vi "GOOP_Utility_IsLibVI.vi"(7 "KeepClassOpen(False)":bool, 8 "error in (no error)":errorcluster, 10 "ProjectItem":refnum<vi>, 11 "Object":u64) -> (0 "error out":errorcluster, 1 "ClassItem(If Found)":refnum<vi>, 2 "LibProvider":string, 3 "Is Lib VI?":bool)   [LabVIEW 2014]
uses:
  <resource>/Framework/Providers/Open_GDS/ClassProviders/Common/LvLib_class/GDSLvLib_LibTypeSettingNames.ctl
  <resource>/Framework/Providers/Open_GDS/ClassProviders/Provider_LvNativeClass/LvNativeProviderName.ctl
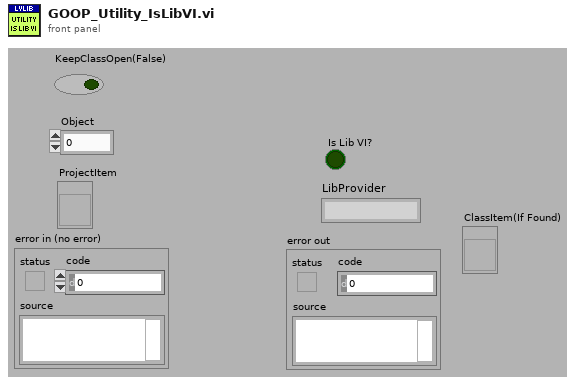
[diagram p1: front panel]
types:
  T1 = typedef "LvNativeProviderName.ctl" = enum16{"Endevo LabVIEW Native"}
  T2 = typedef "GDSLvLib_LibTypeSettingNames.ctl" = enum16{"EndevoGOOP_LibProvider", "EndevoGOOP_TemplateUsed", "EndevoGOOP_TemplateVersion", "EndevoGOOP_PlugIns", "EndevoGOOP_ConnectorPanePattern"}
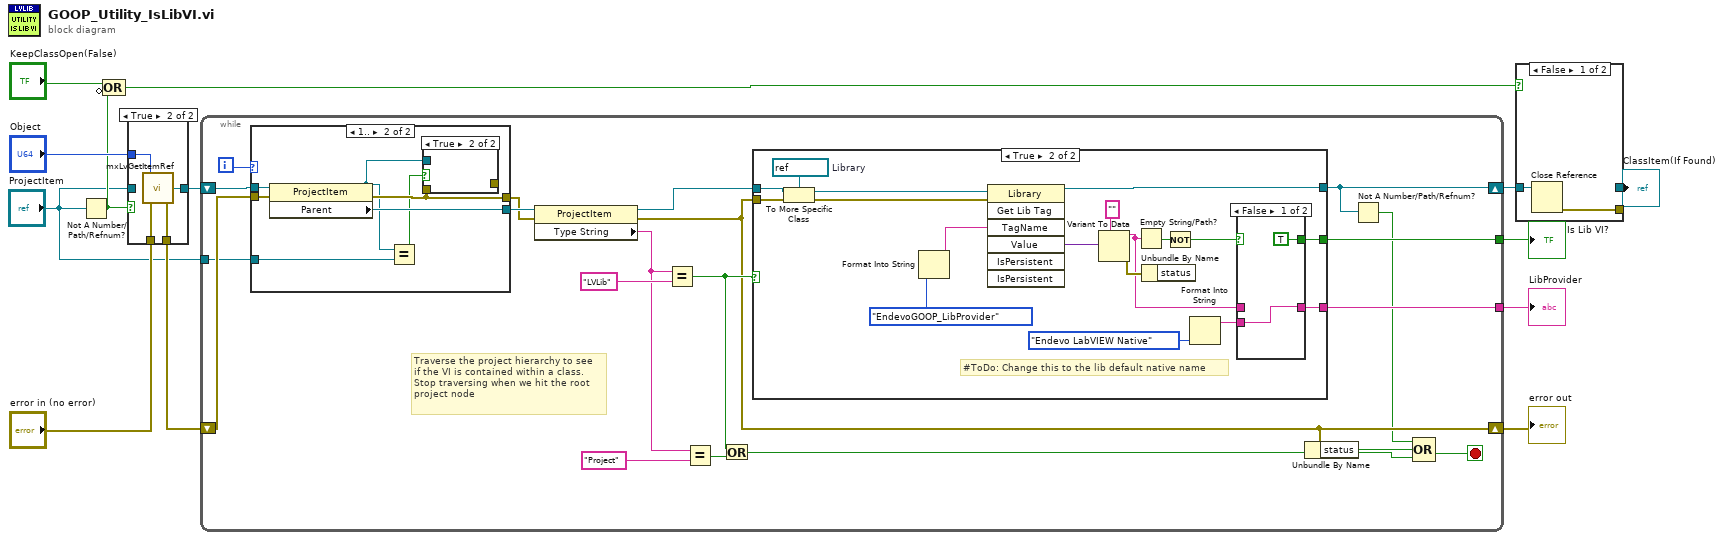
[diagram p0: block diagram]
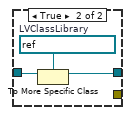
[diagram p3: hidden frame]
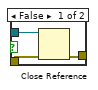
[diagram p5: hidden frame]
diagram:
  n1 = Not A Number/Path/Refnum?(number/path/refnum="ProjectItem") -> (NaN/Path/Refnum?=w2:bool)
  n2 = Compound Arithmetic op=OR("KeepClassOpen(False)", invert w2) -> (w3:bool)
  n3 = case shown="True" w2 {
    tunnel: "Object" -> [_ w19]
    tunnel: [w14 w18] -> w12
    tunnel: "error in (no error)" -> [w15 w17]
    tunnel: [w15 w16] -> w8
    tunnel: "ProjectItem" -> [w14 _]
    frame False {
    }
    frame True {
      n4 = call <resource>:"mxLvGetItemRef.vi"("Item"=w19, "error in"=w17) -> ("Item Refnum"=w18:refnum<vi>, "error out"=w16:errorcluster)  [unwired: 1 out]
    }
  }
  n5 = while {
    shift-right: [w25] -> w6
    shift-left: w12 -> [w37]
    tunnel: [w31] -> w11
    tunnel: [w30] -> w9
    shift-right: [w26] -> w7
    shift-left: w8 -> [w29]
    tunnel: "ProjectItem" -> [w20]
    i -> [w27]
    stop <- w21 stop-if-true
    # "Traverse the project hierarchy to see\nif the VI is contained within a class.\nStop traversing when we hit the root\nproject node"
    n6 = case shown="1.." w27 {
      tunnel: [w40 w48] -> w38
      tunnel: w37 -> [w40 w47]
      tunnel: w29 -> [w41 w46]
      tunnel: [w41 w45] -> w28
      tunnel: w20 -> [_ w43]
      frame Default {
      }
      frame 1.. {
        n7 = property class="ProjectItem"(reference=w47, error in=w46) -> (reference out=w44:refnum<vi>, error out=w45:errorcluster, "Parent"=w48:refnum<vi>)
        n8 = Equal?(x=w44, y=w43) -> (x = y?=w42:bool)
        n9 = case shown="True" w42 {
          tunnel: w45 -> [w51 _]
          tunnel: w44 -> [w50 _]
          tunnel: [w49 _] -> _
          frame False {
            n10 = Close Reference(reference=w50, error in (no error)=w51) -> (error out=w49:errorcluster)
          }
          frame True {
          }
        }
      }
    }
    n11 = property class="ProjectItem"(reference=w38, error in=w28) -> (reference out=w32:refnum<vi>, error out=w26:errorcluster, "Type String"=w35:string)
    n12 = Equal?(x=w35, y="LVLib") -> (x = y?=w33:bool)
    n13 = Equal?(x=w35, y="Project") -> (x = y?=w34:bool)
    n14 = Or(x=w33, y=w34) -> (x .or. y?=w22:bool)
    n15 = case shown="True" w33 {
      tunnel: w32 -> [w52 w70]
      tunnel: [w52 w68] -> w25
      tunnel: [_ w57] -> w31
      tunnel: [_ w56] -> w30
      tunnel: w26 -> [_ w64]
      frame False {
      }
      frame True {
        w69 = refnum<vi> refnum  # Library
        # "#ToDo: Change this to the lib default native name"
        n16 = To More Specific Class(target class=w69, reference=w70, error in=w64) -> (specific class reference=w54:refnum<vi>, error out=w53:errorcluster)
        n17 = Format Into String(GDSLvLib_LibTypeSettingNames."EndevoGOOP_LibProvider" ("ClassTypeSettingNames")) -> (resulting string=w63:string)  [unwired: 3 in, 1 out]
        n18 = invoke class="Library" method="Get Lib Tag"(reference=w54, error in=w53, "TagName"=w63) -> (reference out=w68:refnum<vi>, "Value"=w67:variant)  [unwired: 4 in, 5 out]
        n19 = Variant To Data(type="", Variant=w67) -> (data=w58:string, error out=w61:errorcluster)  [unwired: 1 in]
        n20 = Empty String/Path?(string/path=w58) -> (empty?=w65:bool)
        n21 = Unbundle By Name(w61) -> ()  [unwired: 1 out]
        n22 = Not(x=w65) -> (.not. x?=w59:bool)
        n23 = Format Into String(LvNativeProviderName."Endevo LabVIEW Native" ("ProviderName")) -> (resulting string=w55:string)  [unwired: 3 in, 1 out]
        n24 = case shown="False" w59 {
          selector: w59 -> [_ w74]
          tunnel: w58 -> [_ w73]
          tunnel: [TRUE w74] -> w57
          tunnel: [w72 w73] -> w56
          tunnel: w55 -> [w72 _]
          frame False {
          }
          frame True {
          }
        }
      }
    }
    n25 = Unbundle By Name(w26) -> ("status"=w24:bool)
    n26 = Not A Number/Path/Refnum?(number/path/refnum=w25) -> (NaN/Path/Refnum?=w23:bool)
    n27 = Compound Arithmetic op=OR(w23, w24, w22) -> (w21:bool)
  }
  "Is Lib VI?" <- w11
  "error out" <- w7
  "LibProvider" <- w9
  n28 = case shown="False" w3 {
    tunnel: w6 -> [w76 w78]
    tunnel: [_ w77] -> w4
    tunnel: [w75 _] -> _
    frame False {
      n29 = Close Reference(reference=w76) -> (error out=w75:errorcluster)  [unwired: 1 in]
    }
    frame True {
      w79 = refnum<vi> refnum  # LVClassLibrary
      n30 = To More Specific Class(target class=w79, reference=w78) -> (specific class reference=w77:refnum<vi>)  [unwired: 1 in, 1 out]
    }
  }
  "ClassItem(If Found)" <- w4
